vi "Send-U8-array-fmt0.vi"(7 "Slave address":u8, 8 "error in (no error)":errorcluster, 10 "MOSI Data":u8[](array[numeric]) format="%.0x", 11 "SPI waveform info":T1 {"Last sample" items=["0", "1", "Z", "L", "H", "X", "T", "V"]}) -> (0 "error out":errorcluster, 3 "SPI waveform info out":T1 {"Last sample" items=["0", "1", "Z", "L", "H", "X", "T", "V"]})   [LabVIEW 2016, in "SPIVI.lvlib"]
uses:
  <userlib>/SPI Digital Waveform/_Typedefs/Waveform info-fmt0.ctl
  <userlib>/SPI Digital Waveform/_Typedefs/Timing-ticks-fmt0.ctl
  <userlib>/SPI Digital Waveform/_Typedefs/Data signals.ctl
  <userlib>/SPI Digital Waveform/_Polymorphics/Interpret Data-U8.vi
  <userlib>/SPI Digital Waveform/_Polymorphics/Add First Bit-fmt0.vi
  <userlib>/SPI Digital Waveform/_Polymorphics/Add Middle Bit-fmt0.vi
  <userlib>/SPI Digital Waveform/_Polymorphics/Add Last Bit-fmt0.vi
  <userlib>/SPI Digital Waveform/_Polymorphics/Add CS Idle Time-fmt0.vi
  SPIVI.lvlib
  <userlib>/SPI Digital Waveform/SDW.lvlib
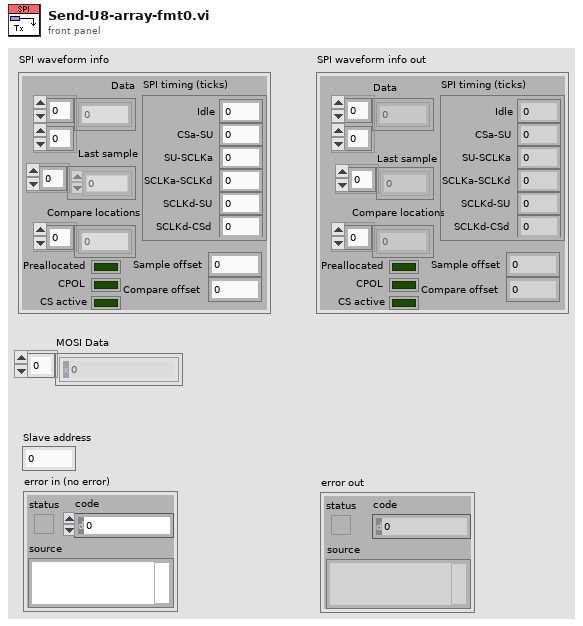
[diagram p1: front panel]
types:
  T1 = typedef "SDW.lvlib/Waveform info-fmt0.ctl" = cluster{"Data":u8[][], "Last sample":u8[], "Preallocated":bool, "Sample offset":u64, "Compare offset":u64, "Compare locations":u64[], "SPI timing (ticks)":T2, "CPOL":bool, "CS active":bool}
  T2 = typedef "SDW.lvlib/Timing-ticks-fmt0.ctl" = cluster{"Idle":i32, "CSa-SU":i32, "SU-SCLKa":i32, "SCLKa-SCLKd":i32, "SCLKd-SU":i32, "SCLKd-CSd":i32}
  T3 = typedef "SDW.lvlib/Data signals.ctl" = u8
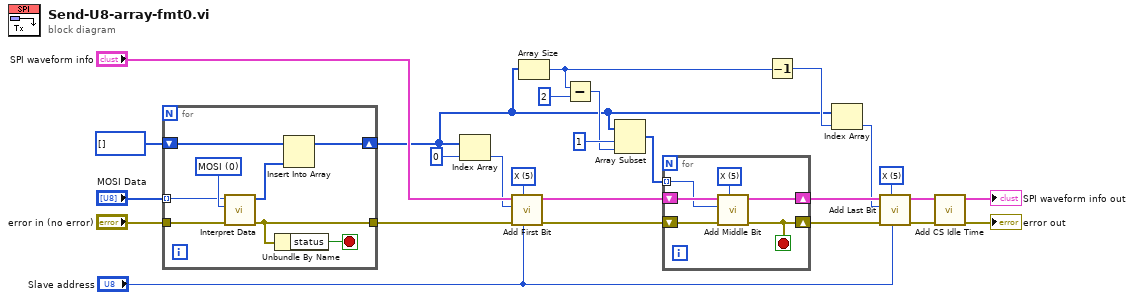
[diagram p0: block diagram]
diagram:
  w6 = u8 5 items=["0", "1", "Z", "L", "H", "X", "T", "V"] ("Expected MISO state")
  w7 = u8 5 items=["0", "1", "Z", "L", "H", "X", "T", "V"] ("Expected MISO state")
  n1 = for {
    tunnel: "MOSI Data" -> [w33] mode=indexing
    shift-right: [w28] -> w1
    shift-left: u8[] [] ("Array of Bits") -> [w30]
    tunnel: "error in (no error)" -> [w32]
    tunnel: [w31] -> w2
    stop <- w27 stop-if-true
    w34 = T3 0 items=["MOSI", "MISO"] ("Data signal")
    n2 = call-poly <userlib>:"Interpret Data.vi"("error in (no error)"=w32, "Data signal"=w34, "Raw data"=w33) -> ("error out"=w31:errorcluster, "Array of Bits"=w29:u8[])  [unwired: 7 out]
    n3 = Unbundle By Name(w31) -> ("status"=w27:bool)
    n4 = Insert Into Array(array=w30, new element=w29) -> (w28:u8[])  [unwired: 1 in]
  }
  n5 = Index Array(array=w1, index=0) -> (element=w17:u8)
  n6 = call-poly <userlib>:"Add First Bit.vi"("Slave address"="Slave address", "Expected MISO state"=w7, "error in (no error)"=w2, "MOSI state"=w17, "SPI waveform info"="SPI waveform info") -> ("error out"=w23:errorcluster, "SPI waveform info out"=w26:T1)  [unwired: 5 out]
  n7 = Array Size(array=w1) -> (size(s)=w13:i32)
  n8 = Subtract(x=w13, y=2) -> (x-y=w15:i32)
  n9 = Array Subset(array=w1, index=1, length=w15) -> (w14:u8[])
  n10 = for {
    shift-right: [w39] -> w25
    shift-left: w26 -> [w40]
    shift-right: [w37] -> w22
    shift-left: w23 -> [w38]
    tunnel: w14 -> [w36] mode=indexing
    stop <- w37 stop-if-true
    w35 = u8 5 items=["0", "1", "Z", "L", "H", "X", "T", "V"] ("Expected MISO state")
    n11 = call-poly <userlib>:"Add Middle Bit.vi"("Expected MISO state"=w35, "error in (no error)"=w38, "MOSI state"=w36, "SPI waveform info"=w40) -> ("error out"=w37:errorcluster, "SPI waveform info out"=w39:T1)  [unwired: 6 out]
  }
  n12 = Decrement(x=w13) -> (x-1=w8:i32)
  n13 = Index Array(array=w1, index=w8) -> (element=w12:u8)
  n14 = call-poly <userlib>:"Add Last Bit.vi"("Slave address"="Slave address", "Expected MISO state"=w6, "error in (no error)"=w22, "MOSI state"=w12, "SPI waveform info"=w25) -> ("error out"=w21:errorcluster, "SPI waveform info out"=w24:T1)  [unwired: 5 out]
  n15 = call-poly <userlib>:"Add CS Idle Time.vi"("error in (no error)"=w21, "SPI waveform info"=w24) -> ("error out"=→"error out":errorcluster, "SPI waveform info out"=→"SPI waveform info out":T1)  [unwired: 8 out]
